vi "Arduino_FindPaths.vi"(8 "error in (no error)":errorcluster, 11 "Arduino In":T1={"Java"=path "/Applications/Arduino.app/Contents/Java", "Packages"=path "/Users/crogers/Library/Arduino15/packages", "folder"=path "", "serial"="", "Console"=""}) -> (0 "error out":errorcluster, 1 "temp code file":path, 2 "Name":string="Code", 3 "Arduino In out":T1)   [LabVIEW 2020]
uses:
  Arduino.ctl
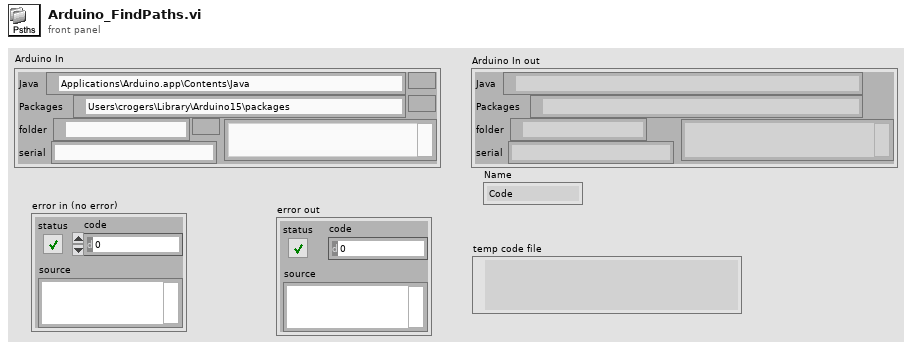
[diagram p1: front panel]
types:
  T1 = typedef "Arduino.ctl" = cluster{"Java":path, "Packages":path, "folder":path, "serial":string, "Console":string}
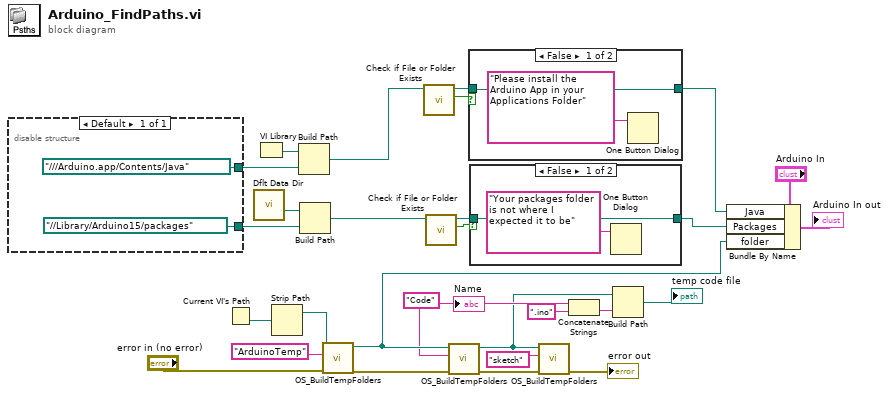
[diagram p0: block diagram]
diagram:
  w17 = "Code" ("Name")
  n1 = disable-structure shown="Default" {
    disable-tunnel: [path "../../../Arduino.app/Contents/Java"] -> w26
    disable-tunnel: [path "../../Library/Arduino15/packages"] -> w25
    frame Enabled {
    }
  }
  n2 = Current VI's Path() -> (path=w2:path)
  n3 = call <vilib>:"Dflt Data Dir.vi"() -> ("App:Default Data Directory"=w24:path)
  n4 = VI Library() -> (path=w4:path)
  n5 = Strip Path(path=w2) -> (stripped path=w3:path)  [unwired: 1 out]
  n6 = Build Path(base path=w4, name or relative path=w26) -> (appended path=w10:path)
  n7 = Build Path(base path=w24, name or relative path=w25) -> (appended path=w9:path)
  n8 = call "OS_BuildTempFolders.vi"("error in (no error)"="error in (no error)", "name"="ArduinoTemp" ("name or relative path"), "path"=w3) -> ("error out"=w13:errorcluster, "appended path"=w20:path)  [unwired: 7 in]
  n9 = call <vilib>:"Check if File or Folder Exists.vi"("path"=w10) -> ("file or folder exists?"=w23:bool, "dup path"=w5:path)  [unwired: 8 in, 1 out]
  n10 = call <vilib>:"Check if File or Folder Exists.vi"("path"=w9) -> ("file or folder exists?"=w11:bool, "dup path"=w8:path)  [unwired: 8 in, 1 out]
  n11 = call "OS_BuildTempFolders.vi"("error in (no error)"=w13, "name"=w17, "path"=w20) -> ("error out"=w21:errorcluster, "appended path"=w15:path)  [unwired: 7 in]
  n12 = case shown="False" w23 {
    tunnel: [w31 w33] -> w6
    tunnel: w5 -> [w31 w33]
    frame False {
      n13 = One Button Dialog(message="Please install the Arduino App in your Applications Folder") -> ()  [unwired: 1 in, 1 out]
    }
    frame True {
    }
  }
  n14 = case shown="False" w11 {
    tunnel: [w34 w36] -> w7
    tunnel: w8 -> [w34 w36]
    frame False {
      n15 = One Button Dialog(message="Your packages folder is not where I expected it to be") -> ()  [unwired: 1 in, 1 out]
    }
    frame True {
    }
  }
  n16 = call "OS_BuildTempFolders.vi"("error in (no error)"=w21, "name"="sketch" ("name or relative path"), "path"=w15) -> ("error out"=→"error out":errorcluster)  [unwired: 7 in, 1 out]
  n17 = Concatenate Strings(w17, ".ino" ("string")) -> (w18:string)
  n18 = Build Path(base path=w15, name or relative path=w18) -> (appended path=→"temp code file":path)
  n19 = Bundle By Name(cluster="Arduino In", "Java"=w6, "Packages"=w7, "folder"=w20) -> (→"Arduino In out":T1)
  "Name" <- w17
